vi "TCP Multiple Connections - Server.vi"() -> ()   [LabVIEW 2019]
doc: "This is the TCP server VI that supports multiple connections from client VIs."
uses:
  controls/TCP Multiple Connections Data.ctl
  controls/TCP Multiple Connections State.ctl
panel:
  in  "Data":T1
  in  "Stop":bool
  out "Current Data":dbl
  out "# of Connections":i32
  # "Overview: Demonstrates the use of the TCP functions to initialize a TCP server that can send data to multiple client VIs.\nInstructions:\n1. Run the VI.\n2. Open TCP Multiple Connections - Client 1.vi and follow the instructions on its front panel.\n3. Open TCP Multiple Connections - Client 2.vi and follow the instructions on its front panel.\n4. Click Stop to stop the VI."
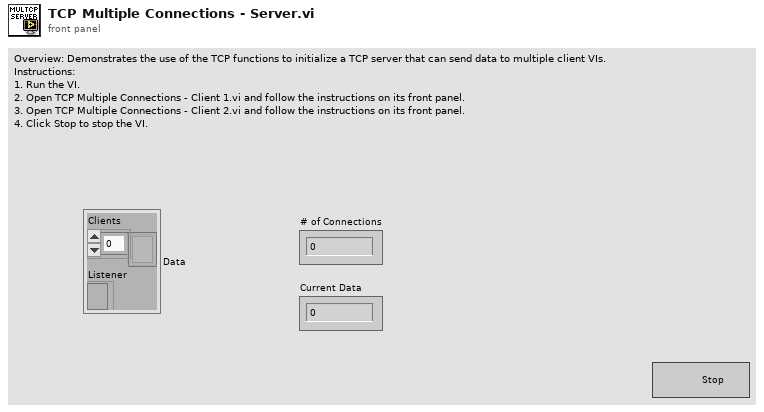
[diagram p1: front panel]
types:
  T1 = typedef "TCP Multiple Connections Data.ctl" = cluster{"Clients":refnum<k5>[], "Listener":refnum<k5>}
  T2 = typedef "TCP Multiple Connections State.ctl" = enum16{"Initialize", "Status Check", "Send Data", "Stop"}
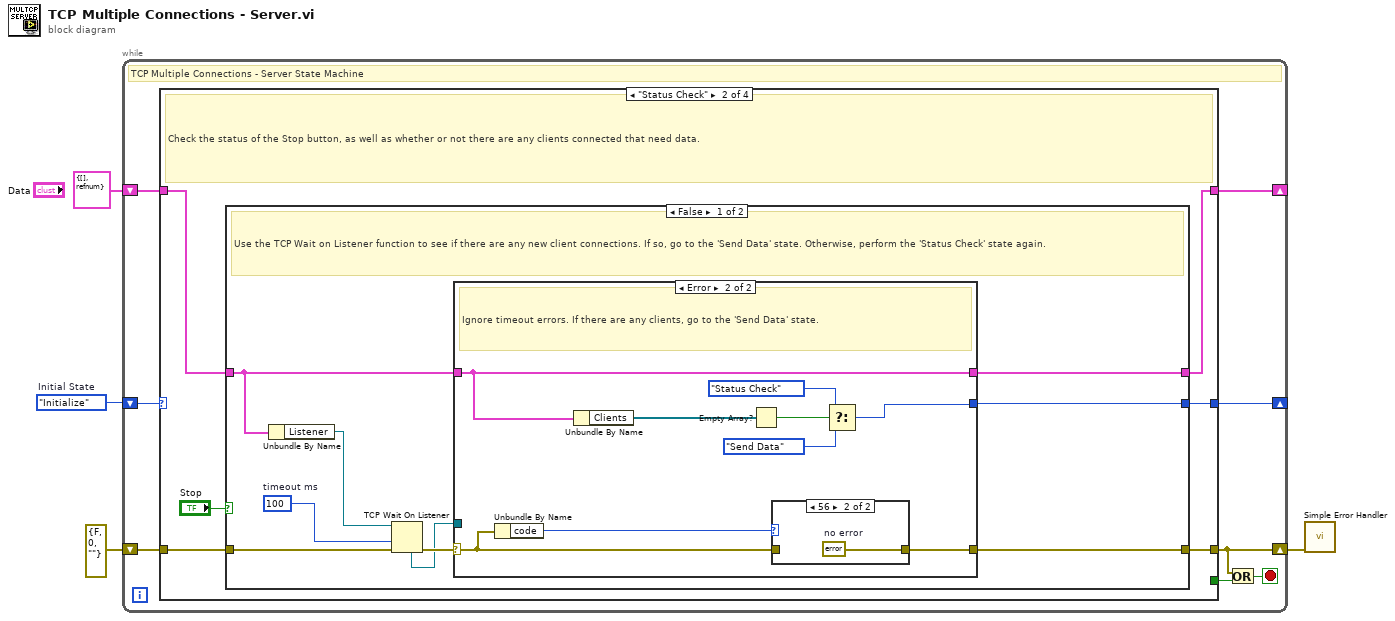
[diagram p0: block diagram]
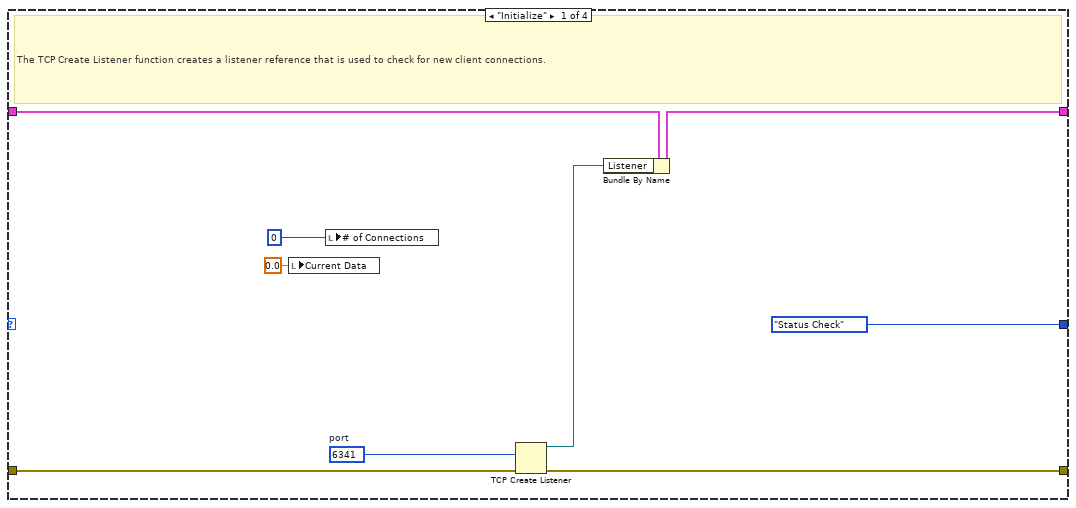
[diagram p2: hidden frame]
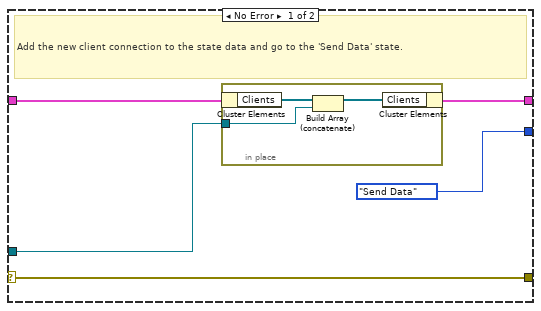
[diagram p3: hidden frame]
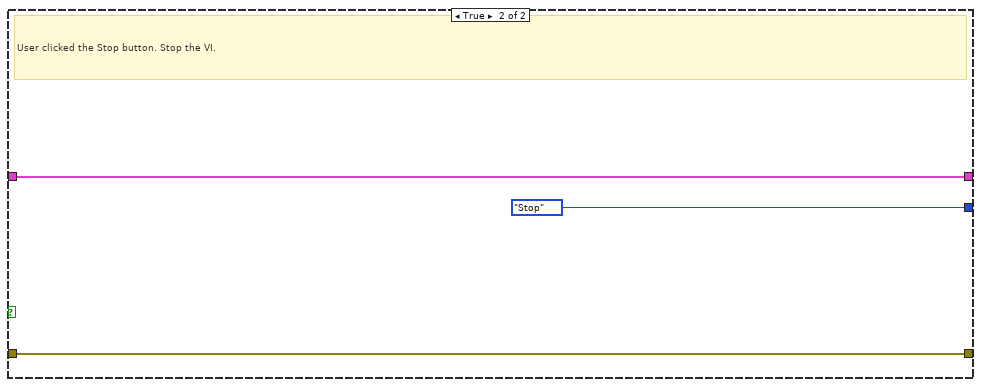
[diagram p5: hidden frame]
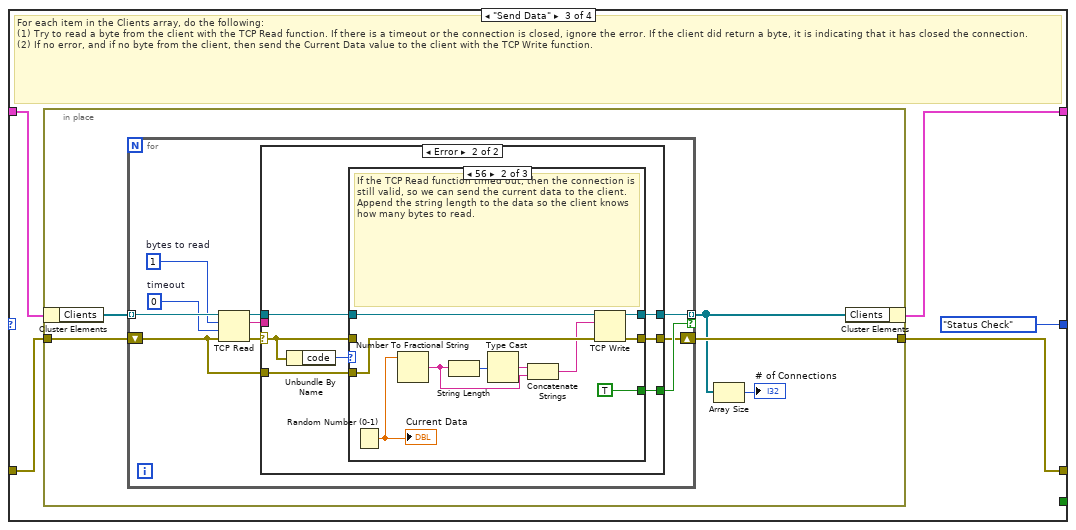
[diagram p6: hidden frame]
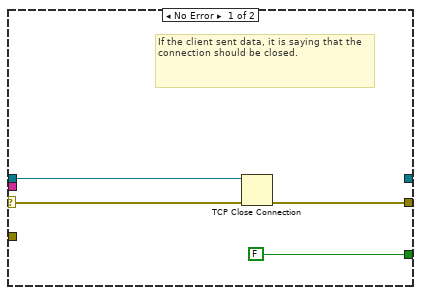
[diagram p7: hidden frame]
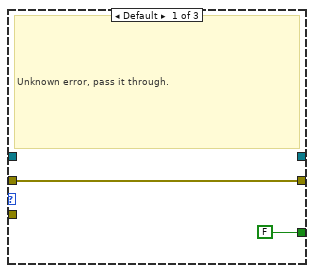
[diagram p8: hidden frame]
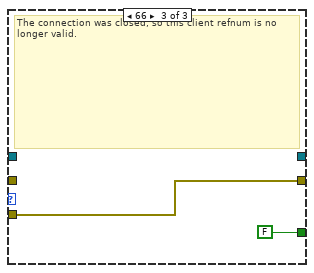
[diagram p9: hidden frame]
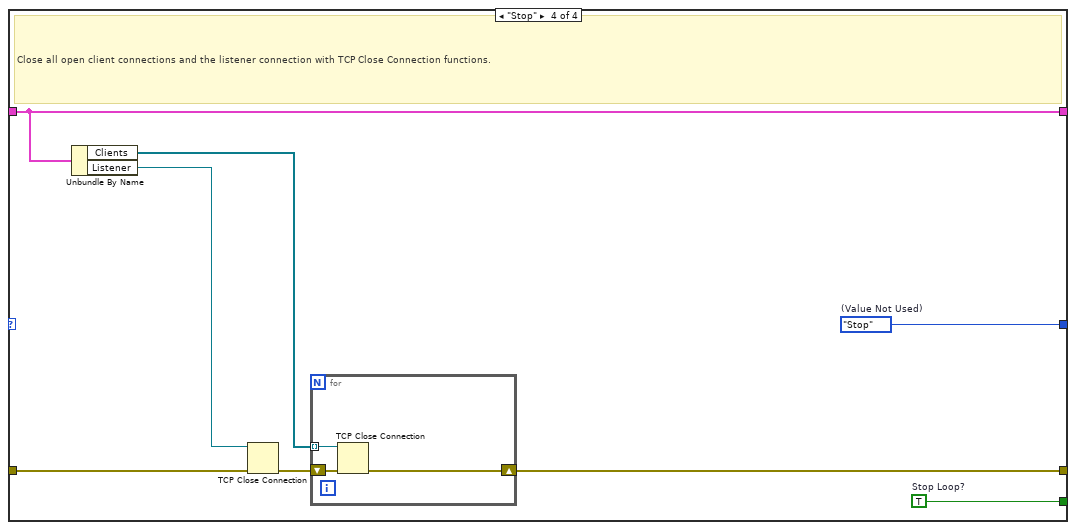
[diagram p10: hidden frame]
diagram:
  w4 = TCP_Multiple_Connections_State."Initialize"  # Initial State
  n1 = while {
    shift-right: [w11] -> _
    shift-left: w4 -> [w12]
    shift-right: [w9] -> _
    shift-left: T1 {"Clients"=[], "Listener"=refnum} ("Data") -> [w10]
    shift-right: [w5] -> w1
    shift-left: errorcluster {"status"=FALSE, "code"=0, "source"=""} ("error constant") -> [w8]
    stop <- w6 stop-if-true
    # "TCP Multiple Connections - Server State Machine"
    n2 = case shown="\"Status Check\"" w12 {
      tunnel: [TCP_Multiple_Connections_State."Status Check" ("States") w27 TCP_Multiple_Connections_State."Status Check" ("States") w104] -> w11
      tunnel: [_ _ _ w111] -> w7
      tunnel: w10 -> [w19 w23 w61 w110]
      tunnel: [w18 w22 w60 w110] -> w9
      tunnel: w8 -> [w21 w26 w63 w109]
      tunnel: [w20 w25 w62 w107] -> w5
      frame "Initialize" {
        w16 = u16 6341  # port
        # "The TCP Create Listener function creates a listener reference that is used to check for new client connections."
        n3 = local write "Current Data"(0.0 ("Current Data")) -> ()
        n4 = local write "# of Connections"(0 ("Number of Client Connections")) -> ()
        n5 = TCP Create Listener(8:w21, 10:w16) -> (0:w20:errorcluster, 3:w17:refnum<k5>)  [unwired: 4 out]
        n6 = Bundle By Name(cluster=w19, "Listener"=w17) -> (w18:T1)
      }
      frame "Status Check" {
        # "Check the status of the Stop button, as well as whether or not there are any clients connected that need data."
        n7 = case shown="False" "Stop" {
          tunnel: [w36 TCP_Multiple_Connections_State."Stop" ("States")] -> w27
          tunnel: w26 -> [w35 w58]
          tunnel: [w28 w58] -> w25
          tunnel: w23 -> [w31 w57]
          tunnel: [w30 w57] -> w22
          frame False {
            w34 = 100  # timeout ms
            # "Use the TCP Wait on Listener function to see if there are any new client connections. If so, go to the 'Send Data' state. Otherwise, perform the 'Status Check' state again."
            n8 = Unbundle By Name(w31) -> ("Listener"=w29:refnum<k5>)
            n9 = TCP Wait On Listener(8:w35, 9:w34, 11:w29) -> (0:w33:errorcluster, 4:w32:refnum<k5>)  [unwired: 4 out]
            n10 = case shown="Error" w33 {
              selector: w33 -> [w39 w53]
              tunnel: [TCP_Multiple_Connections_State."Send Data" ("States") w47] -> w36
              tunnel: w32 -> [w40 _]
              tunnel: w31 -> [w41 w50]
              tunnel: [w38 w50] -> w30
              tunnel: [w39 w51] -> w28
              frame No Error {
                # "Add the new client connection to the state data and go to the 'Send Data' state."
                n11 = in-place {
                  in-place-border: w40 -> [w42]
                  n12 = in-place-cluster #1(w41) -> ("Clients"=w44:refnum<k5>[])
                  n13 = Build Array (concatenate)(w44, w42) -> (w43:refnum<k5>[])
                  n14 = in-place-cluster #1("Clients"=w43) -> (w38:T1)
                }
              }
              frame Error {
                # "Ignore timeout errors. If there are any clients, go to the 'Send Data' state."
                n15 = Unbundle By Name(w53) -> ("code"=w52:i32)
                n16 = Unbundle By Name(w50) -> ("Clients"=w49:refnum<k5>[])
                n17 = Empty Array?(array=w49) -> (empty?=w48:bool)
                n18 = case shown="56" w52 {
                  tunnel: w53 -> [w54 _]
                  tunnel: [w54 w55] -> w51
                  frame Default {
                  }
                  frame 56 {
                    w55 = errorcluster {"status"=FALSE, "code"=0, "source"=""}  # no error
                  }
                }
                n19 = Select(t=TCP_Multiple_Connections_State."Status Check" ("States"), s=w48, f=TCP_Multiple_Connections_State."Send Data" ("States")) -> (s? t:f=w47:T2)
              }
            }
          }
          frame True {
            # "User clicked the Stop button. Stop the VI."
          }
        }
      }
      frame "Send Data" {
        # "For each item in the Clients array, do the following:\n(1) Try to read a byte from the client with the TCP Read function. If there is a timeout or the connection is closed, ignore the error. If the client did return a byte, it is indicating that it has closed the connection.\n(2) If no error, and if no byte from the client, then send the Current Data value to the client with the TCP Write function."
        n20 = in-place {
          in-place-border: w63 -> [w68]
          in-place-border: [w67] -> w62
          n21 = in-place-cluster #2(w61) -> ("Clients"=w65:refnum<k5>[])
          n22 = for {
            tunnel: w65 -> [w78] mode=indexing
            shift-right: [w70] -> w67
            shift-left: w68 -> [w69]
            tunnel: [w72] -> w64 mode=indexing if=w71
            w75 = 0  # timeout
            w76 = 1  # bytes to read
            n23 = TCP Read(connection ID=w78, bytes to read=w76, error in (no error)=w69, 9:w75) -> (connection ID out=w77:refnum<k5>, data out=w73:string, error out=w74:errorcluster)  [unwired: 1 out]
            n24 = case shown="Error" w74 {
              selector: w74 -> [w81 w88]
              tunnel: w77 -> [w82 w85]
              tunnel: w73 -> [_ _]
              tunnel: [_ w83] -> w72
              tunnel: [FALSE w84] -> w71
              tunnel: [w79 w87] -> w70
              tunnel: w69 -> [_ w86]
              frame No Error {
                # "If the client sent data, it is saying that the connection should be closed."
                # "If the client sent data, it is saying that the connection should be closed."
                n25 = TCP Close Connection(connection ID=w82, error in (no error)=w81) -> (error out=w79:errorcluster)  [unwired: 2 out]
              }
              frame Error {
                # "Ignore connection closed and timeout errors"
                n26 = Unbundle By Name(w88) -> ("code"=w89:i32)
                n27 = case shown="56" w89 {
                  tunnel: w88 -> [w91 _ _]
                  tunnel: [w91 w101 w103] -> w87
                  tunnel: w86 -> [_ w97 w103]
                  tunnel: w85 -> [_ w100 _]
                  tunnel: [FALSE TRUE FALSE] -> w84
                  tunnel: [_ w99 _] -> w83
                  frame Default {
                    # "Unknown error, pass it through."
                  }
                  frame 56 {
                    # "If the TCP Read function timed out, then the connection is still valid, so we can send the current data to the client. Append the string length to the data so the client knows how many bytes to read."
                    n28 = Random Number (0-1)() -> (number: 0 to 1=w96:dbl)
                    "Current Data" <- w96
                    n29 = Number To Fractional String(number=w96) -> (F-format string=w93:string)  [unwired: 3 in]
                    n30 = String Length(string=w93) -> (length=w94:i32)
                    n31 = Type Cast(x=w94) -> (*(type *) &x=w95:string)  [unwired: 1 in]
                    n32 = Concatenate Strings(w95, w93) -> (w92:string)
                    n33 = TCP Write(connection ID=w100, data in=w92, error in (no error)=w97) -> (connection ID out=w99:refnum<k5>, error out=w101:errorcluster)  [unwired: 2 out]
                  }
                  frame 66 {
                    # "The connection was closed, so this client refnum is no longer valid."
                  }
                }
              }
            }
          }
          n34 = Array Size(array=w64) -> (size(s)=→"# of Connections":i32)
          n35 = in-place-cluster #2("Clients"=w64) -> (w60:T1)
        }
      }
      frame "Stop" {
        w104 = TCP_Multiple_Connections_State."Stop"  # (Value Not Used)
        w111 = TRUE  # Stop Loop?
        # "Close all open client connections and the listener connection with TCP Close Connection functions."
        n36 = Unbundle By Name(w110) -> ("Clients"=w108:refnum<k5>[], "Listener"=w105:refnum<k5>)
        n37 = TCP Close Connection(connection ID=w105, error in (no error)=w109) -> (error out=w106:errorcluster)  [unwired: 1 in, 1 out]
        n38 = for {
          shift-right: [w113] -> w107
          shift-left: w106 -> [w114]
          tunnel: w108 -> [w112] mode=indexing
          n39 = TCP Close Connection(connection ID=w112, error in (no error)=w114) -> (error out=w113:errorcluster)  [unwired: 1 in, 1 out]
        }
      }
    }
    n40 = Or(x=w5, y=w7) -> (x .or. y?=w6:bool)
  }
  n41 = call <vilib>:"Simple Error Handler.vi"("error in (no error)"=w1) -> ()  [unwired: 4 in, 5 out]
